vi "Untitled 22.vi"() -> ()   [LabVIEW 2012]
uses:
  <vilib>/addons/database/Connection.llb/DB Tools Open Connec (Path).vi
  <vilib>/addons/database/NI_Database_API.lvlib
panel:
  out "error out":errorcluster
  out "data":variant[][](array[variant])
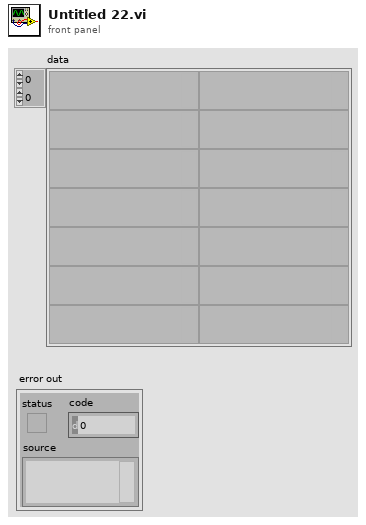
[diagram p1: front panel]
types:
  T1 = typedef "NI_Database_API.lvlib/Conn ObjectReference.ctl" = refnum<k1>
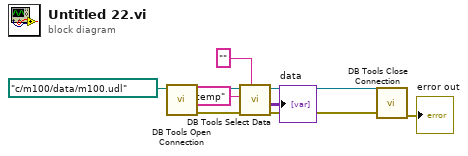
[diagram p0: block diagram]
diagram:
  n1 = call-poly <vilib>:"DB Tools Open Connection.vi"("connection information"=path "c:/m100/data/m100.udl") -> ("error out"=w7:errorcluster, "connection reference"=w8:T1)  [unwired: 7 in]
  n2 = call <vilib>:"DB Tools Select Data.vi"("condition"="", "error in (no error)"=w7, "table"="hot_temp", "connection reference"=w8) -> ("error out"=w5:errorcluster, "data"=→"data":variant[][], "connection reference out"=w6:T1)  [unwired: 2 in]
  n3 = call <vilib>:"DB Tools Close Connection.vi"("error in (no error)"=w5, "connection reference"=w6) -> ("error out"=→"error out":errorcluster)  [unwired: 5 in]
